vi "KB-EMG Input.vi"(7 "Other Message":string, 10 "EMG Iput":string, 11 "Emg":bool) -> (3 "String OutPut":string)   [LabVIEW 2017]
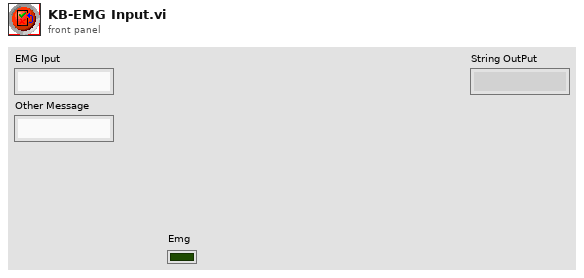
[diagram p1: front panel]
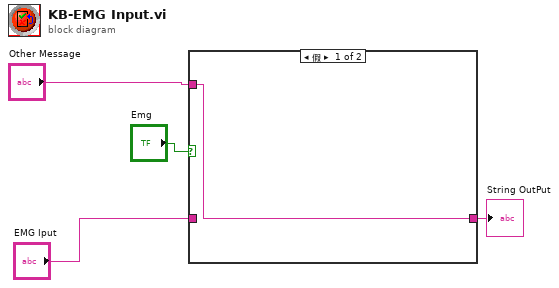
[diagram p0: block diagram]
diagram:
  n1 = case shown="假" "Emg" {
    tunnel: "EMG Iput" -> [_ w6]
    tunnel: [w5 w6] -> w2
    tunnel: "Other Message" -> [w5 _]
    frame False {
    }
    frame True {
    }
  }
  "String OutPut" <- w2
